vi "JSON TO TEMP.vi"(7 "IP":string="192.168.23.100", 8 "error in (no error)":errorcluster, 10 "PORT":dbl=1.0 min=1.0 max=4.0 step=1.0, 11 "MASTER":dbl=1.0 min=1.0 max=10.0 step=1.0) -> (0 "error out":errorcluster, 2 "Thermometer":dbl(slide) scale=0.0..100.0)   [LabVIEW 2024]
uses:
  <vilib>/JDP Science/JSONtext/JSONtext.lvlib
  <userlib>/_OpenG.lib/string/string.llb/openg_string.lvlib
panel:
  out "JSON DATA":string
  # "Thermo data from Smart Conn"
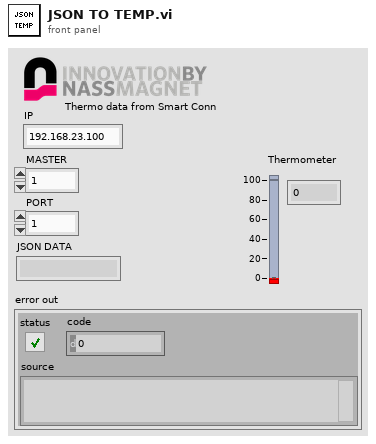
[diagram p1: front panel]
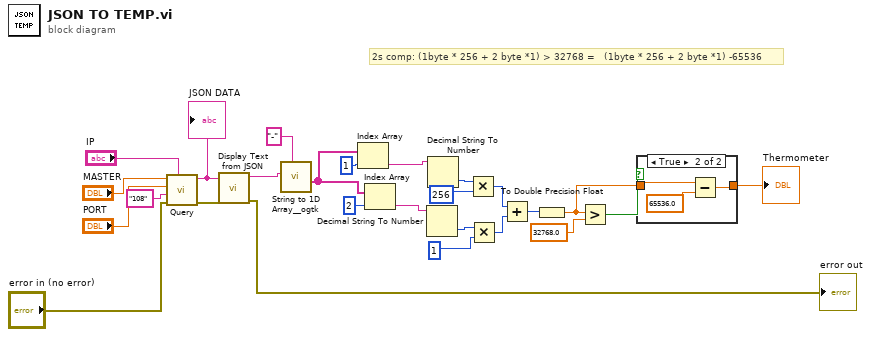
[diagram p0: block diagram]
diagram:
  # "2s comp: (1byte * 256 + 2 byte *1) > 32768 =   (1byte * 256 + 2 byte *1) -65536"
  n1 = call "Query.vi"("IP"="IP", "error in (no error)"="error in (no error)", "PARAMETERS"="108", "PORT"="PORT", "MASTER"="MASTER") -> ("error out"=w18:errorcluster, "JSON data"=w26:string)  [unwired: 5 in]
  "JSON DATA" <- w26
  n2 = call <vilib>:"Display Text from JSON.vi"("error in (no error)"=w18, "Input JSON"=w26) -> ("error out"=→"error out":errorcluster, "Display Text"=w11:string)  [unwired: 7 in, 1 out]
  n3 = call <userlib>:"String to 1D Array__ogtk.vi"("delimiter (Tab)"="-", "string"=w11) -> ("Array of Strings"=w22:string[])  [unwired: 9 in]
  n4 = Index Array(array=w22, index=1) -> (element=w12:string)
  n5 = Index Array(array=w22, index=2) -> (element=w13:string)
  n6 = Decimal String To Number(string=w13) -> (number=w15:i32)  [unwired: 2 in, 1 out]
  n7 = Decimal String To Number(string=w12) -> (number=w9:i32)  [unwired: 2 in, 1 out]
  n8 = Multiply(x=w9, y=u32 256) -> (x*y=w10:u32)
  n9 = Multiply(x=w15, y=u32 1) -> (x*y=w14:u32)
  n10 = Add(x=w10, y=w14) -> (x+y=w5:u32)
  n11 = To Double Precision Float(number=w5) -> (double precision float=w4:dbl)
  n12 = Greater?(x=w4, y=32768.0) -> (0:w2:bool)
  n13 = case shown="True" w2 {
    tunnel: w4 -> [w27 w29]
    tunnel: [w27 w28] -> w3
    frame False {
    }
    frame True {
      n14 = Subtract(x=w29, y=65536.0) -> (x-y=w28:dbl)
    }
  }
  "Thermometer" <- w3
